vi "Host Main.vi"() -> ()   [LabVIEW 2015]
doc: "This application launches and executes the Tag Bus Data framework configuration for the specified target alias. This is a simple example of the framework API functions, but may also be a suitable starting point for a Host UI or Thick Client that is running a local version of the framework."
uses:
  <vilib>/NI/Module Execution Interface/Engine Runtime/Execution States.ctl
  <vilib>/NI/Module Execution Interface/Engine Runtime/Fault.ctl
  <vilib>/NI/Tag Bus Module Framework/runtime/error classification.ctl
  module/configuration/Runtime Implementation.ctl
  <vilib>/NI/Module Execution Interface/Engine Runtime/Engine Runtime Interface.lvclass
  <vilib>/NI/DCAF/Tag Editor Core/Framework Configuration Classes/target runtime/PL_Target Runtime.lvclass
  <vilib>/NI/Tag Bus Module Framework/runtime/TBM module execution interface.lvclass
  module/configuration/E2E Tag Exchange configuration.lvclass
panel:
  out "DCAF Configuration File":path
  in  "Runtime Implementation":T1
  out "engine status":T5(array[cluster])
  in  "stop":bool
  # "Instructions:\n1. Select a Runtime implementation from the drop down selector box\n2. Run the VI - One User Interface will be displayed for each DCAF engine\n3. Manipulate the controls on each UI to verify the tag transfer to the other engine\n    (Controls in the Ouput Section of each UI are linked to the indicators in the \n      Input Section of the other engine's UI)"
  # "View the runtime specific configuration by opening the displayed configuration file in the DCAF\nconfiguration editor (Tools>>DCAF>>Launch Standard Configuration Editor...)"
  # "View the status information for each engine here"
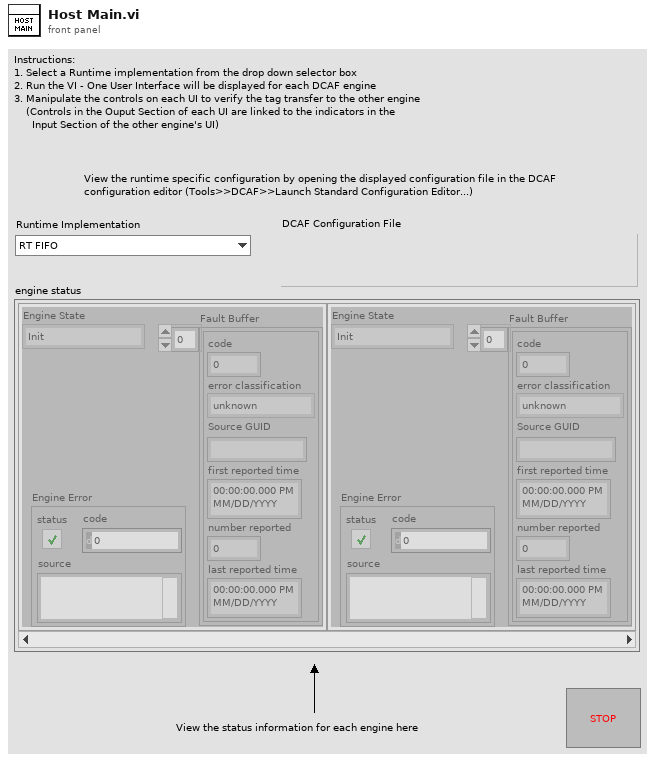
[diagram p1: front panel]
types:
  T1 = typedef "E2E Tag Exchange configuration.lvclass/Runtime Implementation.ctl" = enum16{"RT FIFO", "UDP"}
  T2 = typedef "Engine Runtime Interface.lvclass/Execution States.ctl" = enum16{"Init", "Pre-Operational", "Safe-Operational", "Operational", "Stopped"}
  T3 = typedef "Engine Runtime Interface.lvclass/Fault.ctl" = cluster{"code":i32, "error classification":T4, "Source GUID":string, "first reported time":timestamp, "number reported":u32, "last reported time":timestamp}
  T4 = typedef "TBM module execution interface.lvclass/error classification.ctl" = enum16{"unknown", "none", "trivial", "recoverable", "critical"}
  T5 = cluster{"Engine State":T2, "Fault Buffer":T3[], "Engine Error":errorcluster}[]
  T6 = cluster{"Engine State":T2, "Fault Buffer":T3[], "Engine Error":errorcluster}
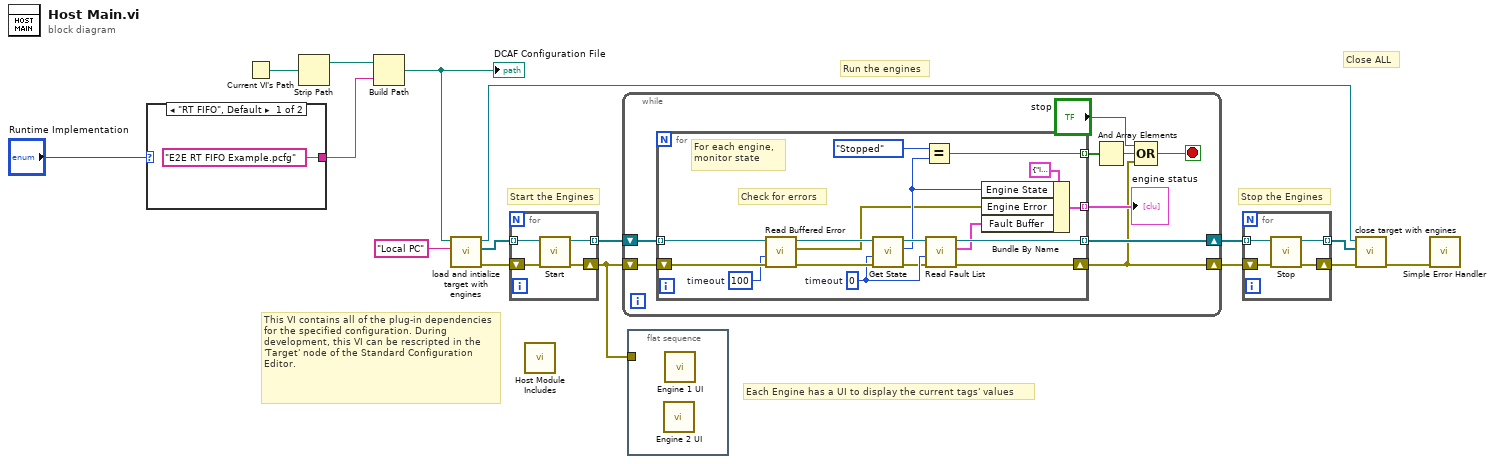
[diagram p0: block diagram]
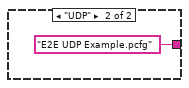
[diagram p2: hidden frame]
diagram:
  # "Each Engine has a UI to display the current tags' values"
  # "Start the Engines"
  # "Close ALL"
  # "Stop the Engines"
  # "This VI contains all of the plug-in dependencies for the specified configuration. During development, this VI can be rescripted in the 'Target' node of the Standard Configuration Editor."
  # "Run the engines"
  n1 = case shown="\"RT FIFO\", Default" "Runtime Implementation" {
    tunnel: ["E2E RT FIFO Example.pcfg" ("target alias") "E2E UDP Example.pcfg" ("target alias")] -> w4
    frame "RT FIFO", Default {
    }
    frame "UDP" {
    }
  }
  n2 = Current VI's Path() -> (path=w5:path)
  n3 = Strip Path(path=w5) -> (stripped path=w6:path)  [unwired: 1 out]
  n4 = Build Path(base path=w6, name or relative path=w4) -> (appended path=w2:path)
  "DCAF Configuration File" <- w2
  n5 = call <vilib>:"load and intialize target with engines.vi"("target alias"="Local PC", "file path"=w2) -> ("error out"=w13:errorcluster, "engine runtime interfaces"=w12:refnum<class "Engine Runtime Interface.lvclass">[], "target runtime"=w10:refnum<class "PL_Target Runtime.lvclass">)  [unwired: 7 in]
  n6 = for {
    tunnel: [w22] -> w16 mode=indexing
    tunnel: w12 -> [w19] mode=indexing
    shift-right: [w21] -> w1
    shift-left: w13 -> [w20]
    n7 = call-dynamic "Start.vi"("error in"=w20, "Engine Runtime Interface in"=w19) -> ("error out"=w21:errorcluster, "Engine Runtime Interface out"=w22:refnum<class "Engine Runtime Interface.lvclass">)  [unwired: 8 in]
  }
  n8 = call "Host Module Includes.vi"() -> ()  [unwired: 12 in]
  n9 = while {
    shift-right: [w29] -> w15
    shift-left: w16 -> [w31]
    shift-right: [w23] -> w14
    shift-left: w1 -> [w30]
    stop <- w27 stop-if-true
    n10 = for {
      tunnel: w31 -> [w48] mode=indexing
      tunnel: [w40] -> w29 mode=indexing
      tunnel: [w43] -> w25 mode=indexing
      shift-right: [w39] -> w23
      shift-left: w30 -> [w47]
      tunnel: [w35] -> w26 mode=indexing
      w38 = 0  # timeout
      w42 = 100  # timeout
      # "For each engine, \nmonitor state"
      # "Check for errors"
      n11 = call-dynamic "Read Buffered Error.vi"("error in"=w47, "timeout in ms (0)"=w42, "Engine Runtime Interface in"=w48) -> ("error out"=w45:errorcluster, "Engine Error"=w33:errorcluster, "Engine Runtime Interface out"=w46:refnum<class "Engine Runtime Interface.lvclass">)  [unwired: 6 in]
      n12 = call-dynamic "Get State.vi"("error in"=w45, "timeout (-1)"=w38, "Engine Runtime Interface in"=w46) -> ("error out"=w32:errorcluster, "Engine State"=w37:T2, "Engine Runtime Interface out"=w41:refnum<class "Engine Runtime Interface.lvclass">)  [unwired: 6 in]
      n13 = Equal?(x=Execution_States."Stopped" ("Engine State"), y=w37) -> (x = y?=w43:bool)
      n14 = call-dynamic "Read Fault List.vi"("error in"=w32, "timeout (-1)"=w38, "Engine Runtime Interface in"=w41) -> ("error out"=w39:errorcluster, "faults"=w36:T3[], "Engine Runtime Interface out"=w40:refnum<class "Engine Runtime Interface.lvclass">)  [unwired: 6 in]
      n15 = Bundle By Name(cluster=T6 {"Engine State"=enum."Init", "Fault Buffer"=[], "Engine Error"={"status"=FALSE, "code"=0, "source"=""}}, "Engine State"=w37, "Engine Error"=w33, "Fault Buffer"=w36) -> (w35:T6)
    }
    "engine status" <- w26
    n16 = And Array Elements(Boolean array=w25) -> (logical AND=w24:bool)
    n17 = Compound Arithmetic op=OR("stop", w24, w23) -> (w27:bool)
  }
  n18 = flat-sequence {
    tunnel: w1 -> [_]
    frame #0 {
      n19 = call "Engine 2 UI.vi"() -> ()  [unwired: 12 in]
      n20 = call "Engine 1 UI.vi"() -> ()  [unwired: 12 in]
    }
  }
  n21 = for {
    tunnel: w15 -> [w52] mode=indexing
    shift-right: [w49] -> w9
    shift-left: w14 -> [w51]
    tunnel: [w50] -> w11 mode=indexing
    n22 = call-dynamic "Stop.vi"("error in"=w51, "Engine Runtime Interface in"=w52) -> ("error out"=w49:errorcluster, "Engine Runtime Interface out"=w50:refnum<class "Engine Runtime Interface.lvclass">)  [unwired: 8 in]
  }
  n23 = call <vilib>:"close target with engines.vi"("error in"=w9, "Engine Runtime Interfaces"=w11, "Target Runtime"=w10) -> ("error out"=w3:errorcluster)  [unwired: 8 in]
  n24 = call <vilib>:"Simple Error Handler.vi"("error in (no error)"=w3) -> ()  [unwired: 4 in, 5 out]
